vi "Process SDL Repeats.vi"(6 "Player":T1, 8 "error in (no error)":errorcluster) -> (0 "error out":errorcluster)   [LabVIEW 2021, in "Main Controller Actor.lvclass"]
uses:
  Main Controller Actor.lvclass
  Ship/Ship.lvclass
  C:/dev/LabVIEW/LabMelee/Source/Application Specific/Element/Element.lvclass
  Ship/Ship.lvclass/Ship.ctl
  Globals.vi
  Control State/Control State.lvclass
  Player.ctl
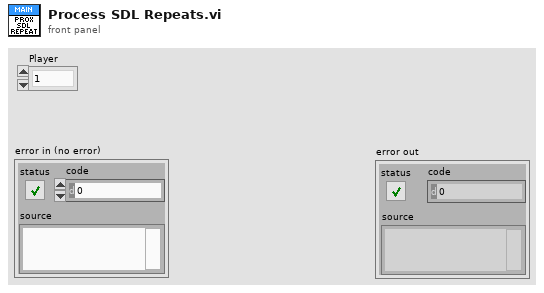
[diagram p1: front panel]
types:
  T1 = typedef "Main Controller Actor.lvclass/Player.ctl" = enum16{"1", "2"}
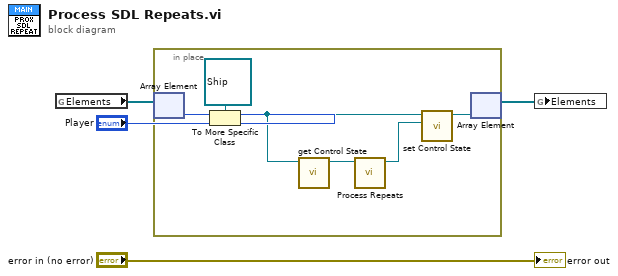
[diagram p0: block diagram]
diagram:
  n1 = global read "Globals.vi" "Elements"() -> (w3:refnum<class "Element.lvclass">[])
  n2 = in-place {
    n3 = in-place-array #1(w3, "Player") -> (w9:refnum<class "Element.lvclass">)
    n4 = To More Specific Class(target class=refnum<class "Ship.lvclass"> refnum ("Ship in"), reference=w9) -> (specific class reference=w7:refnum<class "Ship.lvclass">)  [unwired: 1 in, 1 out]
    n5 = call "get Control State.vi"("Ship in"=w7) -> ("Control State"=w6:refnum<class "Control State.lvclass">)  [unwired: 10 in]
    n6 = call "Process Repeats.vi"("Control State in"=w6) -> ("Control State out"=w5:refnum<class "Control State.lvclass">)  [unwired: 10 in]
    n7 = call-dynamic "set Control State.vi"("Control State"=w5, "Ship in"=w7) -> ("Ship out"=w10:refnum<class "Ship.lvclass">)  [unwired: 9 in]
    n8 = in-place-array #1(w10) -> (w2:refnum<class "Element.lvclass">[])  [unwired: 1 out]
  }
  n9 = global write "Globals.vi" "Elements"(w2) -> ()
  "error out" <- "error in (no error)"
